vi "传感器数据.vi"() -> (3 "传感器读数":T1 {"发的" format="%#.3f"; "拉压力" format="%#.3f"; "一点" format="%#.3f"; "66" format="%#.3f"; "345" format="%#.3f"; "电缸位移" format="%#.3f"; "1" format="%#.3f"; "工装移载位移" format="%#.3f"; "1" format="%#.3f"; "相机结果" format="%#.3f"})   [LabVIEW 2020]
uses:
  Libraries/S7/S7.lvlib
panel:
  out "单精度浮点":sgl
  out "元素":i32
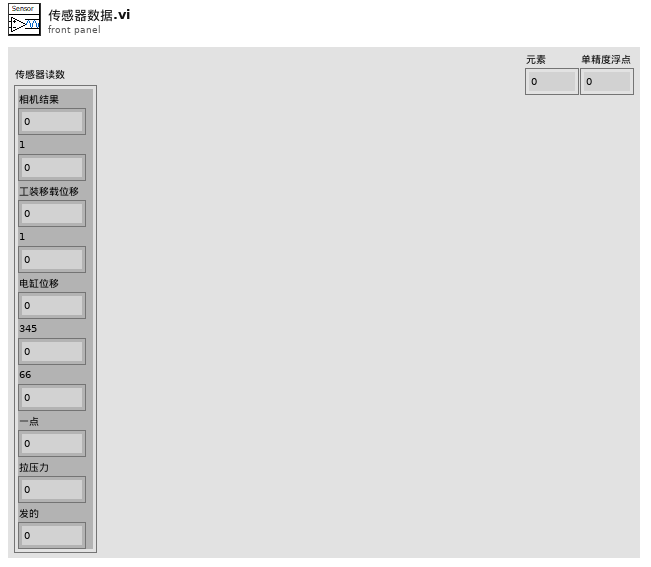
[diagram p1: front panel]
types:
  T1 = cluster{"相机结果":dbl, "1":sgl, "工装移载位移":sgl, "1":sgl, "电缸位移":sgl, "345":sgl, "66":sgl, "一点":sgl, "拉压力":sgl, "发的":sgl}
  T2 = typedef "S7.lvlib/Read_Data (Reply Payload)--cluster.ctl" = cluster{"读取成功":bool, "数据":u32[], "Read_Data_error":errorcluster}
  T3 = cluster{sgl, sgl, sgl, sgl, sgl, sgl, sgl, sgl, sgl, sgl}
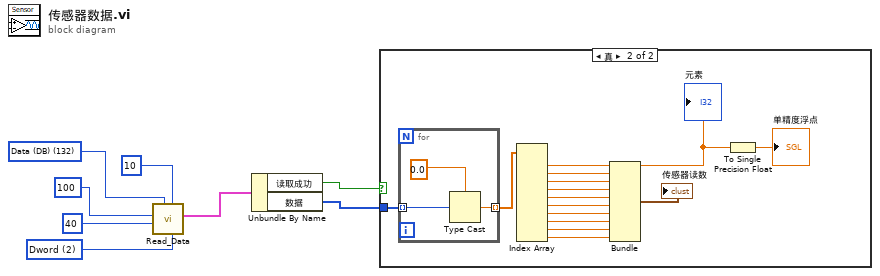
[diagram p0: block diagram]
diagram:
  w5 = u16 2 items=["byte", "word", "Dword"] ("数据类型")
  w6 = u8 132 items=["I/O (P)"=128, "Input (I)"=129, "Output (Q)"=130, "Bit Memory (M)"=131, "Data (DB)"=132, "Instance Data (DI)"=133, "Local Data (L)"=134, "Predecessor Local Data (VL)"=135] ("寄存器类型")
  n1 = call "Read_Data.vi"("数据类型"=w5, "读取长度"=u16 10, "寄存器类型"=w6, "起始地址"=u32 40, "DB #"=u16 100) -> ("Reply Payload"=w3:T2)  [unwired: 4 in, 2 out]
  n2 = Unbundle By Name(w3) -> ("读取成功"=w1:bool, "数据"=w2:u32[])
  n3 = case shown="真" w1 {
    tunnel: w2 -> [_ w22]
    frame False {
    }
    frame True {
      n4 = for {
        tunnel: w22 -> [w25] mode=indexing
        tunnel: [w24] -> w21 mode=indexing
        n5 = Type Cast(type=sgl 0.0, x=w25) -> (*(type *) &x=w24:sgl)
      }
      n6 = Index Array(array=w21) -> (element #1=w12:sgl, element #2=w20:sgl, element #3=w19:sgl, element #4=w18:sgl, element #5=w16:sgl, element #6=w15:sgl, element #7=w14:sgl, element #8=w17:sgl, element #9=w10:sgl, element #10=w9:sgl)  [unwired: 10 in]
      "元素" <- w12
      n7 = Bundle(w12, w20, w19, w18, w16, w15, w14, w17, w10, w9) -> (→"传感器读数":T3)  [unwired: 1 in]
      n8 = To Single Precision Float(number=w12) -> (single precision float=→"单精度浮点":sgl)
    }
  }
